vi "Gyro Acc Dec Back C2Stop.vi"(4 "Threshold to trigger C2":i32=1200, 6 "Ini. Degrees":sgl, 7 "Motor":cluster{"Port":T2, "Port":T2}={"Port"=1, "Port"=2} {"Port" items=["Port A", "Port B", "Port C", "Port D"]; "Port" items=["Port A", "Port B", "Port C", "Port D"]}, 8 "Threshold to De-acc":i32=1000, 9 "De-acc":i32=40, 10 "Acc":i32=80, 11 "EV3 in":T1) -> (3 "EV3 out":T1)   [LabVIEW 2016]
uses:
  <vilib>/NXT/Block Support/NXT_OutputPort.ctl
  <vilib>/NXT/Subs/LVHSConnector.ctl
  <vilib>/NXT/LegoClasses/BrickReference/BrickReference.lvclass
  <vilib>/NXT/Block Support/NXT_InputPort.ctl
  <vilib>/NXT/NXTIO Xnodes/NXTIONodeSubVIs/LEGOResetMotors.vi
  <vilib>/NXT/Dual Mode Library/Motors/Rotation.vi
  <vilib>/NXT/Dual Mode Library/Sensors/EV3_Gyro_Angle.vi
  <vilib>/NXT/Dual Mode Library/Sensors/EV3_Color_Reflect.vi
  <vilib>/NXT/NXTIO Xnodes/NXTIONodeSubVIs/NXTMotorSteeringOn.vi
  <vilib>/NXT/NXTIO Xnodes/NXTIONodeSubVIs/NXTStopMotors.vi
  <vilib>/NXT/Dual Mode Library/Waits/Wait_Num.vi
  <vilib>/NXT/NXTIO Xnodes/NXTIOXNode/NXTIO.xnode
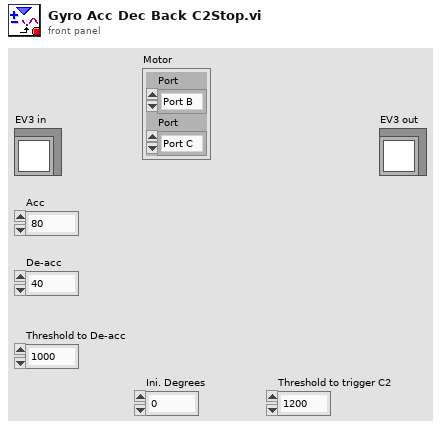
[diagram p1: front panel]
types:
  T1 = typedef "LVHSConnector.ctl" = refnum<class "BrickReference.lvclass">
  T2 = typedef "NXT_OutputPort.ctl" = u8
  T3 = typedef "NXT_InputPort.ctl" = u32
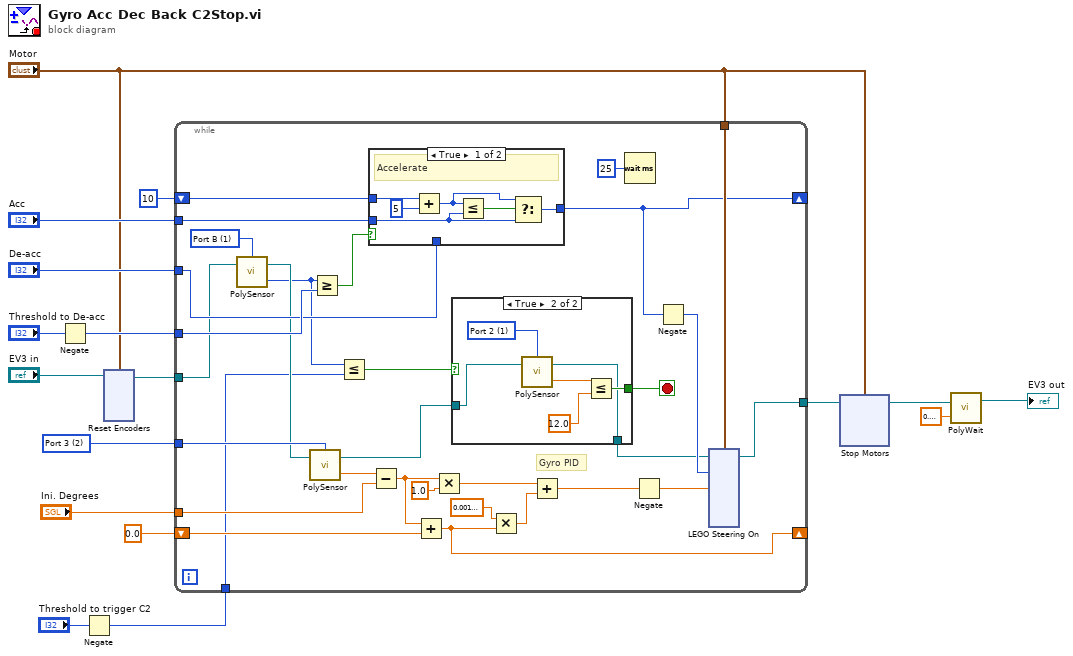
[diagram p0: block diagram]
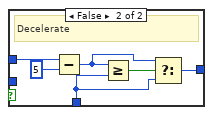
[diagram p3: hidden frame]
diagram:
  w15 = T3 2 items=["Port 1", "Port 2", "Port 3", "Port 4"] ("Port (Gyro)")
  n1 = Negate(x="Threshold to De-acc") -> (-x=w5:i32)
  n2 = Negate(x="Threshold to trigger C2") -> (-x=w6:i32)
  n3 = xnode "Reset Encoders"("Motors"="Motor", "NXT/EV3"="EV3 in") -> ("NXT/EV3"=w12:T1)
  n4 = while {
    tunnel: w12 -> [w29]
    tunnel: w15 -> [w37]
    shift-right: [w45] -> _
    shift-left: sgl 0.0 -> [w46]
    tunnel: "Ini. Degrees" -> [w41]
    tunnel: [w36] -> w8
    tunnel: "Motor" -> [w39]
    shift-right: [w23] -> _
    shift-left: 10 -> [w33]
    tunnel: "De-acc" -> [w30]
    tunnel: "Acc" -> [w32]
    tunnel: w5 -> [w31]
    tunnel: w6 -> [w25]
    stop <- w19 stop-if-true
    w38 = T2 1 items=["Port A", "Port B", "Port C", "Port D"] ("Port (Port A)")
    # "Gyro PID"
    n5 = call-poly <vilib>:"PolySensor.vi"("NXT/EV3"=w29, "Port (Port A)"=w38) -> ("Angle of Rotation"=w26:i32, "NXT/EV3"=w28:T1)  [unwired: 1 in]
    n6 = call-poly <vilib>:"PolySensor.vi"("NXT/EV3"=w28, "Port (Port 1)"=w37) -> ("Degrees"=w48:sgl, "NXT/EV3"=w21:T1)  [unwired: 1 in]
    n7 = Greater Or Equal?(x=w26, y=w31) -> (x >= y?=w27:bool)
    n8 = Less Or Equal?(x=w26, y=w25) -> (x <= y?=w20:bool)
    n9 = case shown="True" w27 {
      tunnel: w32 -> [w57 _]
      tunnel: w33 -> [w60 w66]
      tunnel: [w56 w63] -> w23
      tunnel: w30 -> [_ w62]
      frame True {
        # "Accelerate"
        n10 = Add(x=w60, y=5) -> (x+y=w58:i32)
        n11 = Less Or Equal?(x=w58, y=w57) -> (x <= y?=w59:bool)
        n12 = Select(t=w58, s=w59, f=w57) -> (s? t:f=w56:i32)
      }
      frame False {
        # "Decelerate"
        n13 = Subtract(x=w66, y=5) -> (x-y=w64:i32)
        n14 = Greater Or Equal?(x=w64, y=w62) -> (x >= y?=w65:bool)
        n15 = Select(t=w64, s=w65, f=w62) -> (s? t:f=w63:i32)
      }
    }
    n16 = Subtract(x=w48, y=w41) -> (x-y=w40:sgl)
    n17 = Add(x=w40, y=w46) -> (x+y=w45:sgl)
    n18 = Multiply(x=w40, y=sgl 1.0 ("K_p")) -> (x*y=w43:sgl)
    n19 = case shown="True" w20 {
      tunnel: [_ w52] -> w19
      tunnel: w21 -> [w49 w50]
      tunnel: [w49 w51] -> w18
      frame False {
      }
      frame True {
        w55 = T3 1 items=["Port 1", "Port 2", "Port 3", "Port 4"] ("Port (Port 1)")
        n20 = call-poly <vilib>:"PolySensor.vi"("NXT/EV3"=w50, "Port (Port 1)"=w55) -> ("Scaled Value"=w54:sgl, "NXT/EV3"=w51:T1)  [unwired: 1 in]
        n21 = Less Or Equal?(x=w54, y=sgl 12.0) -> (x <= y?=w52:bool)
      }
    }
    n22 = Multiply(x=sgl 0.001 ("K_i"), y=w45) -> (x*y=w42:sgl)
    n23 = Add(x=w43, y=w42) -> (x+y=w34:sgl)
    n24 = Wait (ms)(milliseconds to wait=u32 25) -> ()  [unwired: 1 out]
    n25 = Negate(x=w34) -> (-x=w22:sgl)
    n26 = Negate(x=w23) -> (-x=w24:i32)
    n27 = xnode "LEGO Steering On"("Steering 1"=w22, "Power 1"=w24, "Motors"=w39, "NXT/EV3"=w18) -> ("NXT/EV3"=w36:T1)
  }
  n28 = xnode "Stop Motors"("Motors"="Motor", "NXT/EV3"=w8) -> ("NXT/EV3"=w2:T1)
  n29 = call-poly <vilib>:"PolyWait.vi"("Time (1 sec)"=sgl 0.2, "NXT/EV3"=w2) -> ("NXT/EV3"=→"EV3 out":T1)  [unwired: 2 in]
